vi "MISC Save Indexed Test File.vi"(0 "Directory Log Path":path, 5 "File Name Root":string, 7 "File Text":string, 9 "Append Mode (Append)":T1=enum."Append", 11 "Error In (no error)":errorcluster, 12 "Iteration":i32, 14 "File Type (T: Data)":bool=TRUE) -> (3 "File Name":string, 4 "Current File Path":path, 15 "Error Out":errorcluster)   [LabVIEW 2011]
uses:
  File IO/Type Defs/FILE Append Mode Enum.ctl
  File IO/Type Defs/FILE Overwrite Warning Enum.ctl
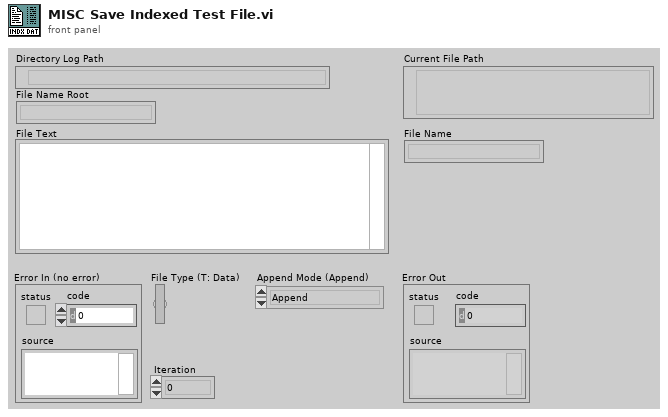
[diagram p1: front panel]
types:
  T1 = typedef "FILE Append Mode Enum.ctl" = enum16{"Overwrite", "Append"}
  T2 = typedef "FILE Overwrite Warning Enum.ctl" = enum16{"Warning", "No Warning"}
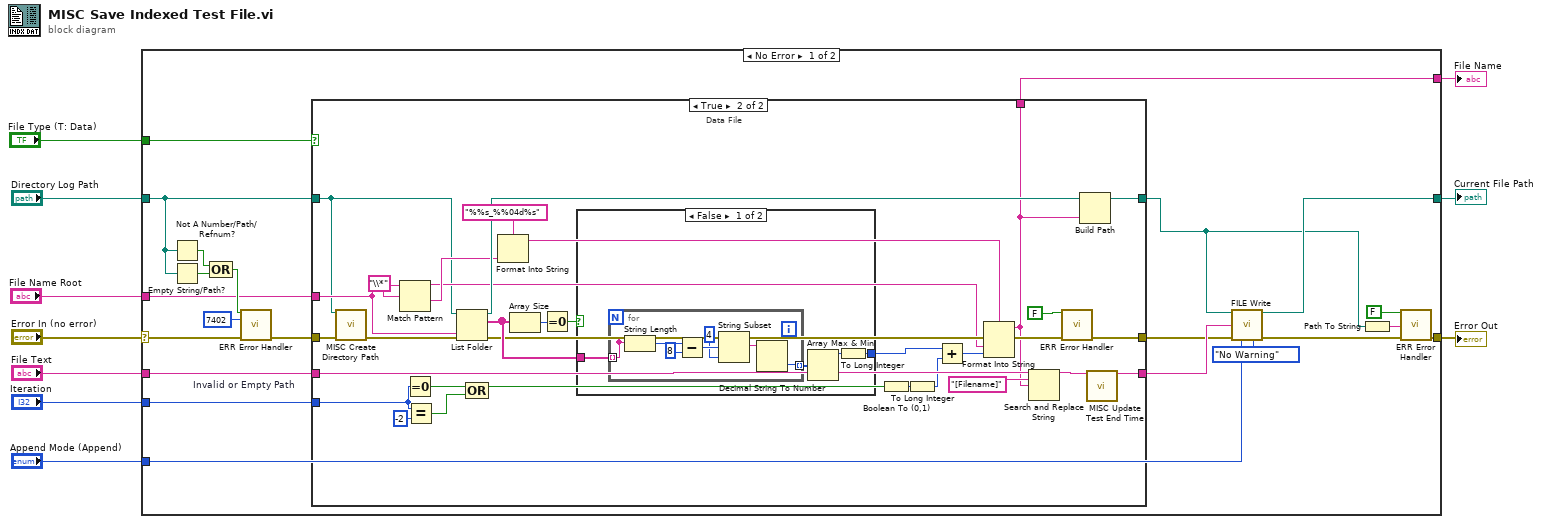
[diagram p0: block diagram]
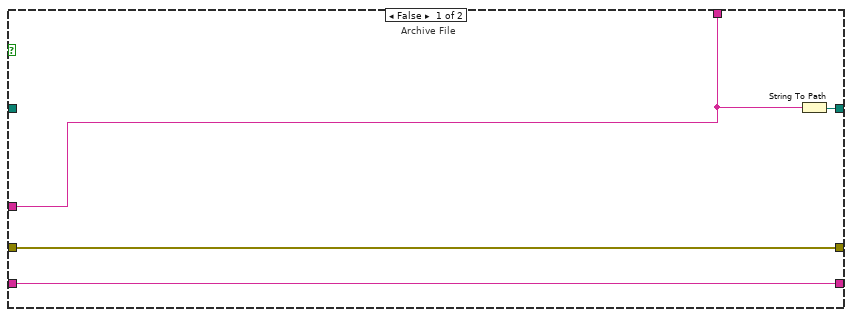
[diagram p2: hidden frame]
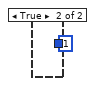
[diagram p3: hidden frame]
diagram:
  n1 = case shown="No Error" "Error In (no error)" {
    selector: "Error In (no error)" -> [w11 w81]
    tunnel: "File Text" -> [w26 _]
    tunnel: "Directory Log Path" -> [w27 w82]
    tunnel: [w21 w81] -> w9
    tunnel: [w19 w82] -> w8
    tunnel: "File Name Root" -> [w15 _]
    tunnel: [w16 _] -> w5
    tunnel: "Iteration" -> [w17 _]
    tunnel: "File Type (T: Data)" -> [w14 _]
    tunnel: "Append Mode (Append)" -> [w13 _]
    frame No Error {
      w28 = 7402  # Invalid or Empty Path
      n2 = Not A Number/Path/Refnum?(number/path/refnum=w27) -> (NaN/Path/Refnum?=w32:bool)
      n3 = Empty String/Path?(string/path=w27) -> (empty?=w31:bool)
      n4 = Compound Arithmetic op=OR(w32, w31) -> (w29:bool)
      n5 = call "ERR Error Handler.vi"("Error Status"=w29, "Error Code"=w28, "Error In (no error)"=w11) -> ("Error Out"=w30:errorcluster)  [unwired: 12 in]
      n6 = case shown="True" w14 {
        tunnel: w30 -> [w35 w41]
        tunnel: w27 -> [_ w40]
        tunnel: w26 -> [w36 w59]
        tunnel: [w36 w37] -> w25
        tunnel: [w35 w53] -> w22
        tunnel: [w34 w52] -> w18
        tunnel: w17 -> [_ w51]
        tunnel: [w33 w42] -> w16
        tunnel: w15 -> [w33 w45]
        frame False {
          # "Archive File"
          n7 = String To Path(string=w33) -> (path=w34:path)
        }
        frame True {
          # "Data File"
          n8 = call "MISC Create Directory Path.vi"("Path"=w40, "Error In (no error)"=w41) -> ("Error Out"=w39:errorcluster)  [unwired: 11 in, 2 out]
          n9 = Match Pattern(string=w45, regular expression="\\*") -> (before substring=w60:string, after substring=w64:string)  [unwired: 1 in, 2 out]
          n10 = Equal To 0?(x=w51) -> (x = 0?=w47:bool)
          n11 = Equal?(x=w51, y=-2) -> (x = y?=w49:bool)
          n12 = List Folder(path=w40, pattern=w45, error in=w39) -> (path out=w68:path, filenames=w66:string[], error out=w61:errorcluster)  [unwired: 1 in, 1 out]
          n13 = Compound Arithmetic op=OR(w47, w49) -> (w48:bool)
          n14 = Format Into String(format string="%%s_%%04d%s" ("Format String"), w64) -> (resulting string=w63:string)  [unwired: 2 in, 1 out]
          n15 = Array Size(array=w66) -> (size(s)=w62:i32)
          n16 = Equal To 0?(x=w62) -> (x = 0?=w67:bool)
          n17 = case shown="False" w67 {
            tunnel: w66 -> [w69 _]
            tunnel: [w70 -1] -> w58
            frame False {
              n18 = for {
                tunnel: w69 -> [w76] mode=indexing
                tunnel: [w79] -> w71 mode=indexing
                n19 = String Length(string=w76) -> (length=w78:i32)
                n20 = Subtract(x=w78, y=8 ("length")) -> (x-y=w75:i32)
                n21 = String Subset(string=w76, offset (0)=w75, length (rest)=4 ("length")) -> (substring=w77:string)
                n22 = Decimal String To Number(string=w77) -> (number=w79:i32)  [unwired: 2 in, 1 out]
              }
              n23 = Array Max & Min(array=w71) -> (max value=w72:i32)  [unwired: 3 out]
              n24 = To Long Integer(number=w72) -> (32bit integer=w70:i32)
            }
            frame True {
            }
          }
          n25 = Boolean To (0,1)(Boolean=w48) -> (0, 1=w57:i16)
          n26 = To Long Integer(number=w57) -> (32bit integer=w56:i32)
          n27 = Add(x=w58, y=w56) -> (x+y=w46:i32)
          n28 = Format Into String(format string=w63, error in=w61, w60, w46) -> (resulting string=w42:string, error out=w54:errorcluster)  [unwired: 1 in]
          n29 = Search and Replace String(input string=w59, search string="[Filename]" ("Search Text"), replace string=w42) -> (result string=w38:string)  [unwired: 5 in, 3 out]
          n30 = call "ERR Error Handler.vi"("Error Status"=FALSE ("Error Flag"), "Error In (no error)"=w54) -> ("Error Out"=w53:errorcluster)  [unwired: 13 in]
          n31 = Build Path(base path=w68, name or relative path=w42) -> (appended path=w52:path)
          n32 = call "MISC Update Test End Time.vi"("Data File"=w38) -> ("New Data File"=w37:string)  [unwired: 14 in]
        }
      }
      n33 = call "FILE Write.vi"("File Path (dialog if empty)"=w18, "Write String"=w25, "Error In (no error)"=w22, "Append/Overwrite (Overwrite)"=w13, "Warn on Overwrite (Warn)"=FILE_Overwrite_Warning_Enum."No Warning" ("warning dialog mode (warn)")) -> ("New File Path"=w19:path, "Error Out"=w23:errorcluster)  [unwired: 9 in]
      n34 = Path To String(path=w18) -> (string=w20:string)
      n35 = call "ERR Error Handler.vi"("Error Status"=FALSE ("Error Flag"), "Cause Of Error"=w20, "Error In (no error)"=w23) -> ("Error Out"=w21:errorcluster)  [unwired: 12 in]
    }
    frame Error {
      (unwired) 0.0
    }
  }
  "Error Out" <- w9
  "Current File Path" <- w8
  "File Name" <- w5
